vi "libssh2_sftp_open.vi"(7 "mode":i32(ring) items=["LIBSSH2_SFTP_S_IRWXU"=448, "LIBSSH2_SFTP_S_IRUSR"=256, "LIBSSH2_SFTP_S_IWUSR"=128, "LIBSSH2_SFTP_S_IXUSR"=64, "LIBSSH2_SFTP_S_IRWXG"=56, "LIBSSH2_SFTP_S_IRGRP"=32, "LIBSSH2_SFTP_S_IWGRP"=16, "LIBSSH2_SFTP_S_IXGRP"=8, "LIBSSH2_SFTP_S_IRWXO"=7, "LIBSSH2_SFTP_S_IROTH"=4, "LIBSSH2_SFTP_S_IWOTH"=2, "LIBSSH2_SFTP_S_IXOTH"=1], 8 "error in (no error)":errorcluster, 9 "flags":u32(ring) format="%x" items=["LIBSSH2_FXF_READ"=1, "LIBSSH2_FXF_WRITE"=2, "LIBSSH2_FXF_APPEND"=4, "LIBSSH2_FXF_CREAT"=8, "LIBSSH2_FXF_TRUNC"=16, "LIBSSH2_FXF_EXCL"=32], 10 "path":string, 11 "sftp":T2) -> (0 "error out":errorcluster, 3 "sftp handle":T1)   [LabVIEW 2013, in "libssh2.lvlib"]
doc: "Open a file handle with default flags and permissions."
uses:
  libssh2.lvlib
  SFTP Refnum.ctl
  SFTP Handle Refnum.ctl
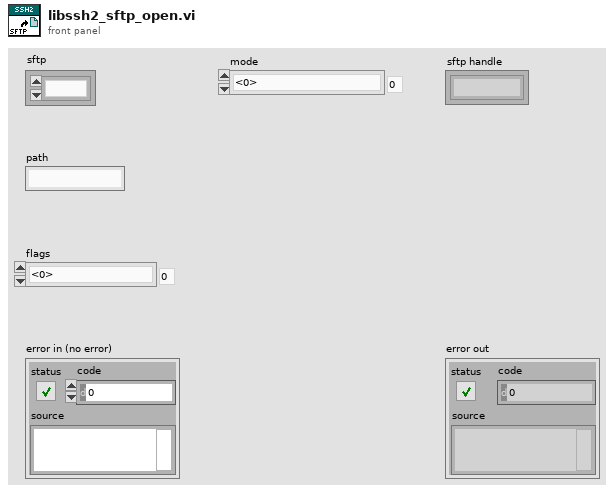
[diagram p1: front panel]
types:
  T1 = typedef "libssh2.lvlib/SFTP Handle Refnum.ctl" = refnum<k1>
  T2 = typedef "libssh2.lvlib/SFTP Refnum.ctl" = refnum<k1>
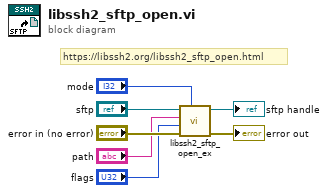
[diagram p0: block diagram]
diagram:
  # "https://libssh2.org/libssh2_sftp_open.html"
  n1 = call "libssh2_sftp_open_ex.vi"("mode"="mode", "error in (no error)"="error in (no error)", "flags"="flags", "filename"="path", "sftp"="sftp") -> ("error out"=→"error out":errorcluster, "sftp handle"=→"sftp handle":T1)  [unwired: 5 in]
